vi "Test REF Configuration.vi"(8 "error in (no error)":errorcluster, 11 "Instrument.Lockin in":refnum<class "Instrument.Lockin.lvclass">) -> (0 "error out":errorcluster, 3 "Instrument.Lockin out":refnum<class "Instrument.Lockin.lvclass">)   [LabVIEW 2016]
uses:
  src/Instrument.Lockin/Instrument.Lockin.lvclass
  src/Instrument.Lockin/Typedefs/REF-cluster.ctl
  src/Instrument.Lockin/Typedefs/REF_f-array.ctl
  src/Instrument.Lockin/Typedefs/REF_phi-array.ctl
  src/Instrument.Lockin/Typedefs/REF_Channel-Numeric.ctl
  src/Instrument.Lockin/Typedefs/REF filter-cluster.ctl
  <userlib>/_OpenG.lib/numeric/numeric.llb/Random Number Within Range - DBL__ogtk.vi
  <vilib>/addons/_JKI Toolkits/Caraya/classes/Assert/Assert Equal Value and Type_Variant.vi
  <vilib>/addons/_JKI Toolkits/Caraya/classes/Assert/Assert Almost Equal_Float.vi
  <userlib>/_OpenG.lib/numeric/numeric.llb/Random Number Within Range - I32__ogtk.vi
  <vilib>/addons/_JKI Toolkits/Caraya/classes/Test/Test.lvclass
  <vilib>/addons/_JKI Toolkits/Caraya/classes/Assert/Assert.lvclass
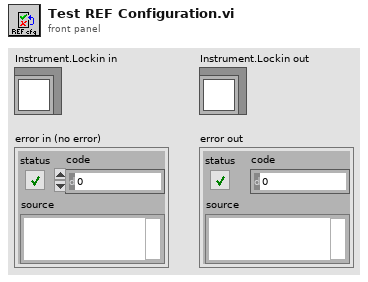
[diagram p1: front panel]
types:
  T1 = typedef "Instrument.Lockin.lvclass/REF filter-cluster.ctl" = cluster{"TC (s)":dbl, "order":i32}
  T2 = typedef "Instrument.Lockin.lvclass/REF_Channel-Numeric.ctl" = i32
  T3 = typedef "Instrument.Lockin.lvclass/REF-cluster.ctl" = cluster{"REF f (Hz)":T4, "REF phi (°)":T5}
  T4 = typedef "Instrument.Lockin.lvclass/REF_f-array.ctl" = dbl[]
  T5 = typedef "Instrument.Lockin.lvclass/REF_phi-array.ctl" = dbl[]
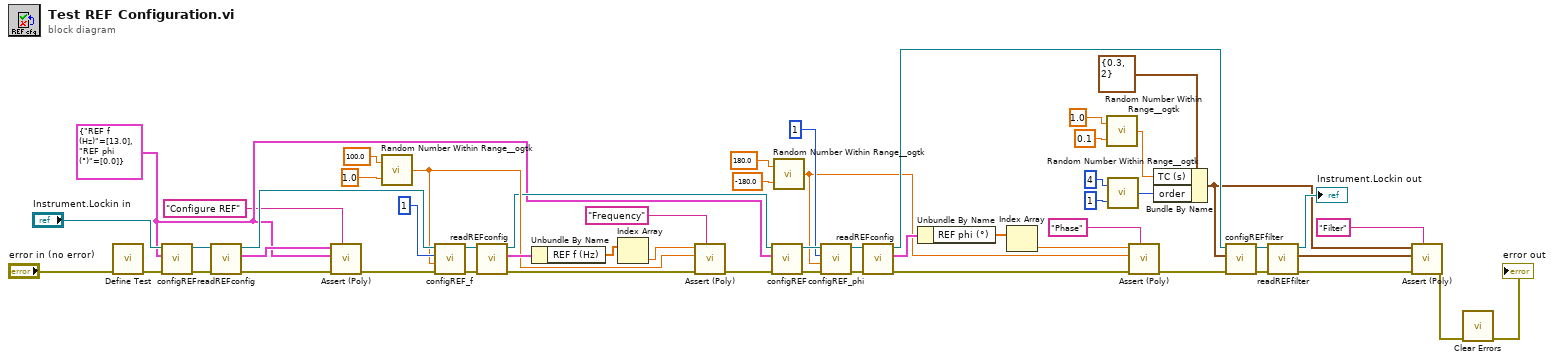
[diagram p0: block diagram]
diagram:
  w27 = T3 {"REF f (Hz)"=[13.0], "REF phi (°)"=[0.0]} ("Channels: Lockin in")
  n1 = call <vilib>:"Define Test.vi"("error in (no error)"="error in (no error)") -> ("error out"=w42:errorcluster)  [unwired: 10 in]
  n2 = call "configREF.vi"("error in (no error)"=w42, "Channels: Lockin in"=w27, "Instrument.Lockin in"="Instrument.Lockin in") -> ("error out"=w46:errorcluster, "Instrument.Lockin out"=w45:refnum<class "Instrument.Lockin.lvclass">)  [unwired: 7 in]
  n3 = call "readREFconfig.vi"("error in (no error)"=w46, "Instrument.Lockin in"=w45) -> ("error out"=w40:errorcluster, "REFconfig"=w41:T3, "Instrument.Lockin out"=w47:refnum<class "Instrument.Lockin.lvclass">)  [unwired: 7 in]
  n4 = call-poly <vilib>:"Assert (Poly).vi"("Label"="Configure REF", "error in (no error)"=w40, "Y"=w27, "X"=w41) -> ("error out"=w39:errorcluster)  [unwired: 7 in]
  n5 = call-poly <userlib>:"Random Number Within Range__ogtk.vi"("High"=100.0, "Low"=1.0) -> ("Random Number"=w31:dbl)  [unwired: 3 in]
  n6 = call "configREF_f.vi"("error in (no error)"=w39, "Frequency (Hz)"=w31, "REF Channel"=T2 1, "Instrument.Lockin in"=w47) -> ("error out"=w49:errorcluster, "Instrument.Lockin out"=w48:refnum<class "Instrument.Lockin.lvclass">)  [unwired: 6 in]
  n7 = call "readREFconfig.vi"("error in (no error)"=w49, "Instrument.Lockin in"=w48) -> ("error out"=w35:errorcluster, "REFconfig"=w34:T3, "Instrument.Lockin out"=w30:refnum<class "Instrument.Lockin.lvclass">)  [unwired: 7 in]
  n8 = Unbundle By Name(w34) -> ("REF f (Hz)"=w33:T4)
  n9 = Index Array(array=w33) -> (element=w32:dbl)  [unwired: 1 in]
  n10 = call-poly <vilib>:"Assert (Poly).vi"("Label"="Frequency", "error in (no error)"=w35, "Y"=w31, "X"=w32) -> ("error out"=w28:errorcluster)  [unwired: 7 in]
  n11 = call "configREF.vi"("error in (no error)"=w28, "Channels: Lockin in"=w27, "Instrument.Lockin in"=w30) -> ("error out"=w23:errorcluster, "Instrument.Lockin out"=w29:refnum<class "Instrument.Lockin.lvclass">)  [unwired: 7 in]
  n12 = call-poly <userlib>:"Random Number Within Range__ogtk.vi"("High"=180.0, "Low"=-180.0) -> ("Random Number"=w19:dbl)  [unwired: 3 in]
  n13 = call "configREF_phi.vi"("error in (no error)"=w23, "Phase (°)"=w19, "REF Channel"=T2 1, "Instrument.Lockin in"=w29) -> ("error out"=w51:errorcluster, "Instrument.Lockin out"=w50:refnum<class "Instrument.Lockin.lvclass">)  [unwired: 6 in]
  n14 = call "readREFconfig.vi"("error in (no error)"=w51, "Instrument.Lockin in"=w50) -> ("error out"=w18:errorcluster, "REFconfig"=w21:T3, "Instrument.Lockin out"=w52:refnum<class "Instrument.Lockin.lvclass">)  [unwired: 7 in]
  n15 = Unbundle By Name(w21) -> ("REF phi (°)"=w22:T5)
  n16 = Index Array(array=w22) -> (element=w20:dbl)  [unwired: 1 in]
  n17 = call-poly <userlib>:"Random Number Within Range__ogtk.vi"("High"=1.0, "Low"=0.1) -> ("Random Number"=w6:dbl)  [unwired: 3 in]
  n18 = call-poly <userlib>:"Random Number Within Range__ogtk.vi"("High"=4, "Low"=1) -> ("Random Number"=w5:i32)  [unwired: 3 in]
  n19 = call-poly <vilib>:"Assert (Poly).vi"("Label"="Phase", "error in (no error)"=w18, "Y"=w19, "X"=w20) -> ("error out"=w17:errorcluster)  [unwired: 7 in]
  n20 = Bundle By Name(cluster=T1 {"TC (s)"=0.3, "order"=2} ("REF filter"), "TC (s)"=w6, "order"=w5) -> (w4:T1)
  n21 = call "configREFfilter.vi"("error in (no error)"=w17, "REF filter"=w4, "Instrument.Lockin in"=w52) -> ("error out"=w54:errorcluster, "Instrument.Lockin out"=w53:refnum<class "Instrument.Lockin.lvclass">)  [unwired: 7 in]
  n22 = call "readREFfilter.vi"("error in (no error)"=w54, "Instrument.Lockin in"=w53) -> ("error out"=w3:errorcluster, "REF filter"=w13:T1, "Instrument.Lockin out"=→"Instrument.Lockin out":refnum<class "Instrument.Lockin.lvclass">)  [unwired: 7 in]
  n23 = call-poly <vilib>:"Assert (Poly).vi"("Label"="Filter", "error in (no error)"=w3, "Y"=w13, "X"=w4) -> ("error out"=w2:errorcluster)  [unwired: 7 in]
  n24 = call <vilib>:"Clear Errors.vi"("error in (no error)"=w2) -> ("error out"=→"error out":errorcluster)  [unwired: 5 in, 1 out]
